vi "Get AI REF (f) StringsAndValues.vi"(8 "error in (no error)":errorcluster, 11 "Instrument.Lockin in":refnum<class "Instrument.Lockin.lvclass">) -> (0 "error out":errorcluster, 2 "AI REF (f) StringsAndValues":cluster{string, i32}[](array[cluster]), 3 "Instrument.Lockin out":refnum<class "Instrument.Lockin.lvclass">)   [LabVIEW 2016, in "Instrument.Lockin.lvclass"]
uses:
  Instrument.Lockin.lvclass
  Instrument.Lockin.lvclass/Instrument.Lockin.ctl
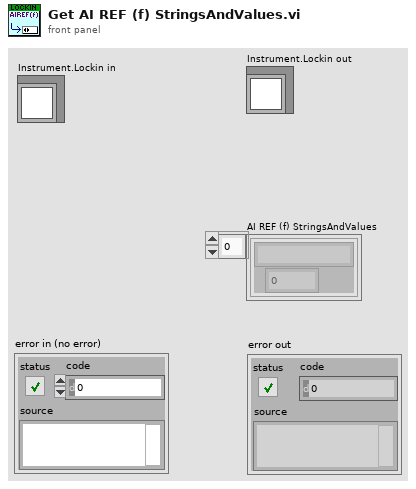
[diagram p1: front panel]
types:
  T1 = typedef "Lockin.DAQ.lvclass/AI.config-array.ctl" = T2[]
  T2 = typedef "Lockin.DAQ.lvclass/AI.config-cluster.ctl" = cluster{"AI.channels":tag, "AI.Coupling":T3, "AI.Range":T4, "input terminal configuration":i32, "DAQ Type":T5}
  T3 = typedef "Lockin.DAQ.lvclass/AI.coupling-enum.ctl" = u16
  T4 = typedef "Lockin.DAQ.lvclass/446xAI-enum.ctl" = enum16{"±0.316", "±1.00", "±3.16", "±10.0", "±31.6", "±42.4"}
  T5 = typedef "Lockin.DAQ.lvclass/DAQType-enum.ctl" = enum16{"None", "USB 4431", "PXI 446x"}
  T6 = typedef "Lockin.DAQ.lvclass/REF-cluster.ctl" = T7[]
  T7 = typedef "Instrument.Lockin.UI.lvclass/REF Channel--Cluster.ctl" = cluster{"Channel":i32, "Frequency":dbl, "Phase":dbl, "TC":dbl, "Order":i32}
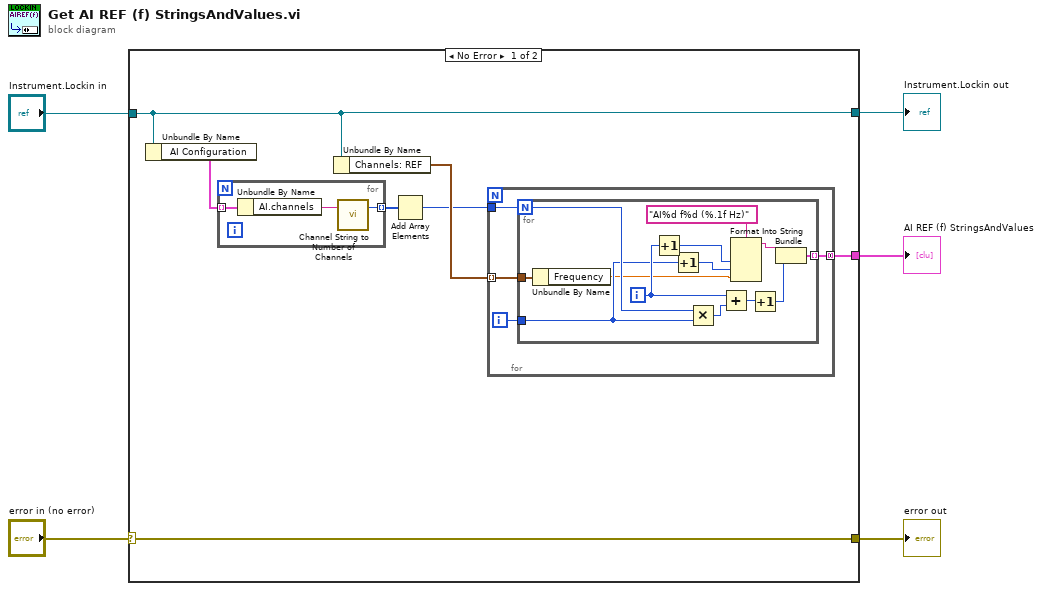
[diagram p0: block diagram]
diagram:
  n1 = case shown="No Error" "error in (no error)" {
    selector: "error in (no error)" -> [w7 w33]
    tunnel: [w10 _] -> w5
    tunnel: "Instrument.Lockin in" -> [w8 w34]
    tunnel: [w8 w34] -> w3
    tunnel: [w7 w33] -> w1
    frame No Error {
      n2 = Unbundle By Name(w8) -> ("AI Configuration"=w12:T1)
      n3 = for {
        tunnel: w12 -> [w15] mode=indexing
        tunnel: [w14] -> w11 mode=indexing
        n4 = Unbundle By Name(w15) -> ("AI.channels"=w13:tag)
        n5 = call "Channel String to Number of Channels.vi"("Channels String"=w13) -> ("# channels"=w14:i32)  [unwired: 2 in]
      }
      n6 = Unbundle By Name(w8) -> ("Channels: REF"=w9:T6)
      n7 = Add Array Elements(numeric array=w11) -> (sum=w6:i32)
      n8 = for {
        tunnel: w9 -> [w17] mode=indexing
        tunnel: [w18] -> w10 mode=concatenating
        tunnel: w6 -> [w16]
        i -> [w19]
        n9 = for {
          N: w16 -> [w27]
          tunnel: [w32] -> w18 mode=indexing
          tunnel: w19 -> [w24]
          tunnel: w17 -> [w22]
          i -> [w25]
          n10 = Unbundle By Name(w22) -> ("Frequency"=w21:dbl)
          n11 = Increment(x=w25) -> (x+1=w20:i32)
          n12 = Increment(x=w24) -> (x+1=w23:i32)
          n13 = Multiply(x=w27, y=w24) -> (x*y=w26:i32)
          n14 = Add(x=w25, y=w26) -> (x+y=w31:i32)
          n15 = Format Into String(format string="AI%d f%d (%.1f Hz)", w20, w23, w21) -> (resulting string=w29:string)  [unwired: 2 in, 1 out]
          n16 = Increment(x=w31) -> (x+1=w28:i32)
          n17 = Bundle(w29, w28) -> (w32:cluster{string, i32})  [unwired: 1 in]
        }
      }
    }
    frame Error {
    }
  }
  "AI REF (f) StringsAndValues" <- w5
  "Instrument.Lockin out" <- w3
  "error out" <- w1
